vi "Connect.vi"(8 "error in":errorcluster, 11 "ThorlabsLabJack in":refnum<class "ThorlabsLabJack.lvclass">) -> (0 "error out":errorcluster, 3 "ThorlabsLabJack out":refnum<class "ThorlabsLabJack.lvclass">)   [LabVIEW 2018, in "ThorlabsLabJack.lvlib" / "ThorlabsLabJack.lvclass"]
uses:
  ThorlabsLabJack.lvclass
  ThorlabsLabJack.lvclass/ThorlabsLabJack.ctl
  C:/Projects/LabVIEW/In-Progress/Chetan Malpure/Axis/Thorlabs LabJack/Drivers/Thorlabs.MotionControl.IntegratedStepperMotorsCLI.dll
  Drivers/Thorlabs.MotionControl.IntegratedStepperMotorsCLI.dll
  LWS_Base/trunk/LabVIEW/PPLs/Configuration/Axis.lvlibp/Axis.lvclass
  C:/Projects/LWS_Base/trunk/LabVIEW/PPLs/Configuration/Axis.lvlibp/Axis.lvclass
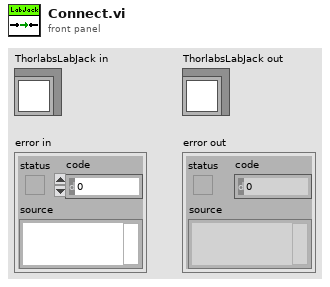
[diagram p1: front panel]
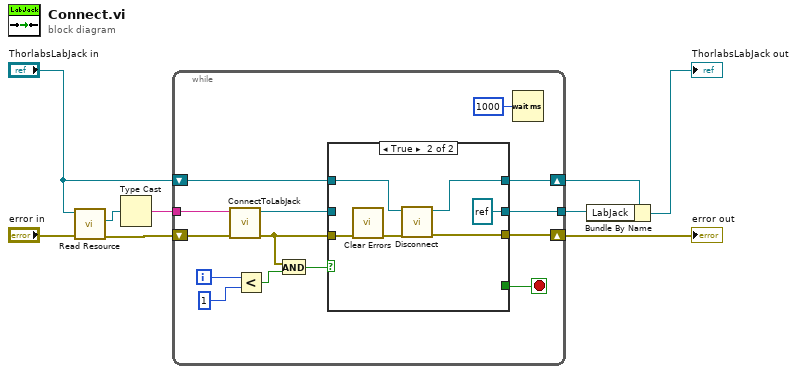
[diagram p0: block diagram]
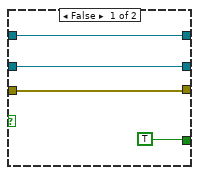
[diagram p2: hidden frame]
diagram:
  n1 = call "Read Resource.vi"("error in"="error in", "Axis in"="ThorlabsLabJack in") -> ("error out"=w4:errorcluster, "Resource"=w8:refnum<visa-resource-name>)  [unwired: 7 in, 1 out]
  n2 = Type Cast(x=w8) -> (*(type *) &x=w9:string)  [unwired: 1 in]
  n3 = while {
    tunnel: w9 -> [w23]
    tunnel: [w12] -> w6
    shift-right: [w15] -> w3
    shift-left: w4 -> [w22]
    shift-right: [w13] -> w1
    shift-left: "ThorlabsLabJack in" -> [w14]
    i -> [w18]
    stop <- w16 stop-if-true
    n4 = call "ConnectToLabJack.vi"("Error In"=w22, "Serial Number"=w23) -> ("Error Out"=w10:errorcluster, "LabJack out"=w17:refnum<k24>)  [unwired: 8 in]
    n5 = Less?(x=w18, y=1) -> (x < y?=w20:bool)
    n6 = And(x=w10, y=w20) -> (x .and. y?=w19:bool)
    n7 = case shown="True" w19 {
      tunnel: w17 -> [w24 _]
      tunnel: w10 -> [w25 w33]
      tunnel: [TRUE _] -> w16
      tunnel: [w25 w31] -> w15
      tunnel: w14 -> [w26 w30]
      tunnel: [w26 w29] -> w13
      tunnel: [w24 refnum<k24> refnum ("LabJack out")] -> w12
      frame False {
      }
      frame True {
        n8 = call <vilib>:"Clear Errors.vi"("error in (no error)"=w33) -> ("error out"=w32:errorcluster)  [unwired: 5 in, 1 out]
        n9 = call-dynamic "Disconnect.vi"("error in"=w32, "ThorlabsLabJack in"=w30) -> ("error out"=w31:errorcluster, "ThorlabsLabJack out"=w29:refnum<class "ThorlabsLabJack.lvclass">)  [unwired: 8 in]
      }
    }
    n10 = Wait (ms)(milliseconds to wait=u32 1000) -> ()  [unwired: 1 out]
  }
  "error out" <- w3
  n11 = Bundle By Name(cluster=w1, "LabJack"=w6) -> (→"ThorlabsLabJack out":refnum<class "ThorlabsLabJack.lvclass">)
